vi "SS2 Live_Download Multiple SS2 Images_v3.vi"(4 "# 8-bit Images (1)":i32=1, 5 "Image ROI Information":T2, 6 "Buffer Size (#8-bit Images)":i32, 7 "SS2 Live Gate Data Q Name":string="SS2 Live Gate Data Q", 8 "Error In":errorcluster, 9 "Image Binning Options":T1={"Use Image Binning"=FALSE, "X Bin"=1, "Y Bin"=1} {"Y Bin" min=1; "X Bin" min=1}, 10 "Display Image":T3, 11 "Device Refnum":refnum<k24>) -> (0 "Error Out":errorcluster, 1 "8-bit Image Count":i32, 2 "Display Image":T3)   [LabVIEW 2019]
uses:
  C:/UCLA Thinkpad Google Drive/LabVIEW 2019 SP1/builds/SS2 Live Distribution/Opal Kelly/C# Wrapper/libFrontPanel-csharp.dll
  Opal Kelly/C# Wrapper/libFrontPanel-csharp.dll
  <vilib>/vision/Image Controls.llb/IMAQ Image.ctl
  SS2 Live_Image ROI Information.ctl
  Phasor/Image Binning Options.ctl
  8f499a87-0ce6-40db-98f3-8f764b7e409e.vi
  8d2e2152-5180-46c7-ad9e-0233ef769053.vi
  <vilib>/Utility/High Resolution Relative Seconds.vi
  <vilib>/Utility/error.llb/Error Cluster From Error Code.vi
  <vilib>/ErrorRing/Error Ring.xnode
  Opal Kelly/C# Wrapper/okFrontPanelC#Wrapper.lvlib
  <vilib>/vision/NI_Vision_Development_Module.lvlib
  Notebook/Notebook.lvlib
  Rich Text Box/Rich Text Box.lvlib
panel:
  out "ReadFromBlockPipeout Error":errorcluster
  out "Activate Trigger Error Out":errorcluster
  out "Timeout error":errorcluster
  out "CPU/8-bit Gate":dbl
  in  "Discard First Image":bool
  in  "Block Size":i32=-1
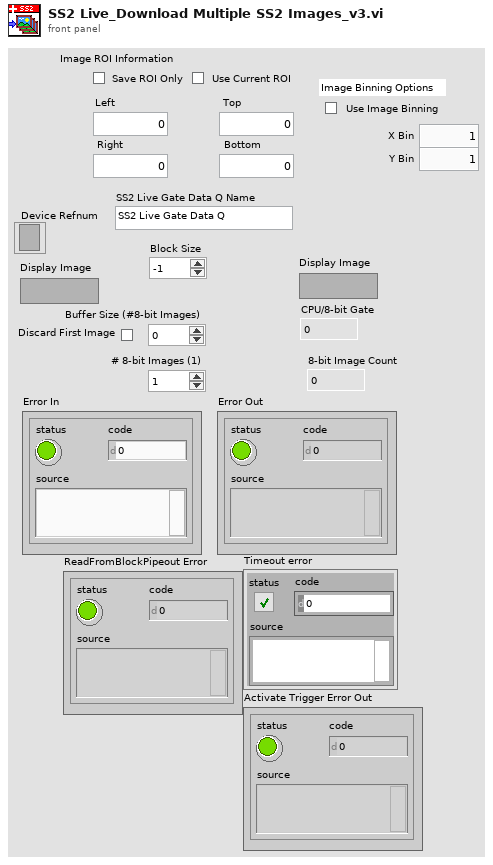
[diagram p1: front panel]
types:
  T1 = typedef "Image Binning Options.ctl" = cluster{"Use Image Binning":bool, "X Bin":i32, "Y Bin":i32}
  T2 = typedef "SS2 Live_Image ROI Information.ctl" = cluster{"Save ROI Only":bool, "Left":u16, "Top":u16, "Right":u16, "Bottom":u16, "Use Current ROI":bool}
  T3 = typedef "IMAQ Image.ctl" = refnum<image>
  T4 = typedef "Image Type" = u32
  T5 = typedef "Rich Text Box.lvlib/Text Formatting.ctl" = cluster{"Font":string, "Text Color":T6, "Text Background Color":T6, "Text Style":enum16{"Regular", "Bold", "Italic", "Underline", "Strikeout"}, "Font Size (Points)":dbl, "Text Alignment":i32}
  T6 = typedef "Rich Text Box.lvlib/Text Colors.ctl" = enum16{"Unchanged", "Black", "Blue", "Gray", "Green", "Red", "White"}
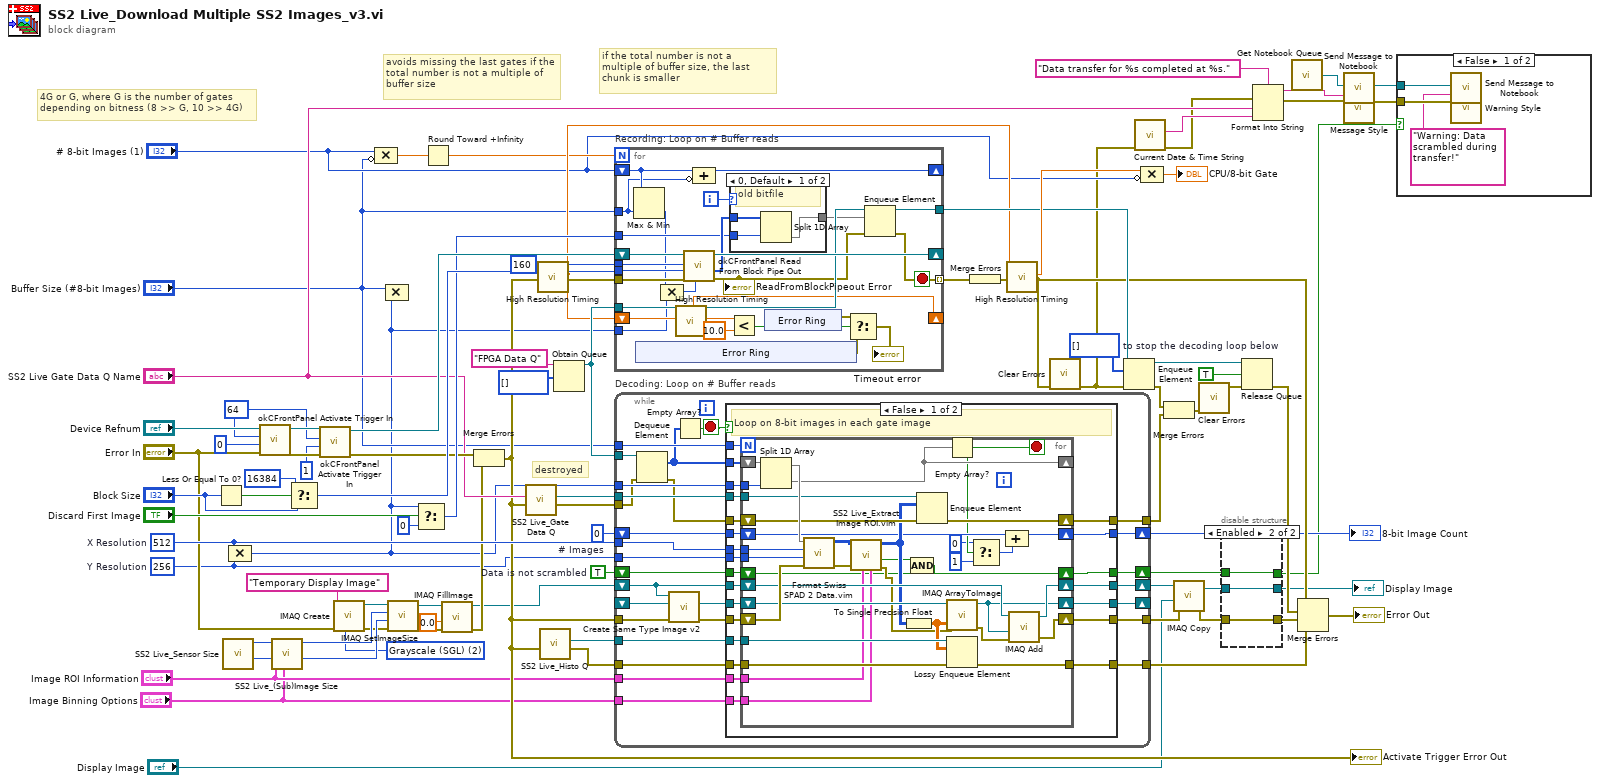
[diagram p0: block diagram]
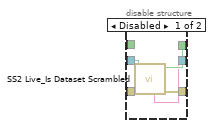
[diagram p2: hidden frame]
diagram:
  w2 = TRUE  # Data is not scrambled
  w21 = T4 2 items=["Grayscale (U8)", "Grayscale (I16)", "Grayscale (SGL)", "Complex (CSG)", "RGB (U32)", "HSL (U32)", "RGB (U64)", "Grayscale (U16)"] ("Image Type")
  w59 = u8[] []  # to stop the decoding loop below
  w61 = 0  # # Images
  w3 = 256  # Y Resolution
  w76 = 512  # X Resolution
  w83 = 64 ("Endpoint Addr")
  # "destroyed"
  # "if the total number is not a multiple of buffer size, the last chunk is smaller"
  # "avoids missing the last gates if the total number is not a multiple of buffer size"
  # "4G or G, where G is the number of gates\ndepending on bitness (8 >> G, 10 >> 4G)"
  n1 = Less Or Equal To 0?(x="Block Size") -> (x <= 0?=w81:bool)
  n2 = call "SS2 Live_Sensor Size.vi"() -> ("Y size"=w22:i32, "X size"=w23:i32)  [unwired: 10 in]
  n3 = Compound Arithmetic op=MULTIPLY(w76, w3) -> (w12:i32)
  n4 = call "okCFrontPanel Activate Trigger In.vi"("Error In"="Error In", "Bit"=0, "Endpoint Addr"=w83, "okCFrontPanel Refnum"="Device Refnum") -> ("Error Out"=w85:errorcluster, "okCFrontPanel Refnum"=w84:refnum<k24>)  [unwired: 6 in]
  n5 = call "SS2 Live_(Sub)Image Size.vi"("Image Binning Options"="Image Binning Options", "Image Information"="Image ROI Information", "# Pixel Y in"=w22, "# Pixel X in"=w23) -> ("# Pixel Y out"=w39:i32, "# Pixel X out"=w40:i32)  [unwired: 6 in]
  n6 = Select(t=16384, s=w81, f="Block Size") -> (s? t:f=w66:i32)
  n7 = call "okCFrontPanel Activate Trigger In.vi"("Error In"=w85, "Bit"=1, "Endpoint Addr"=w83, "okCFrontPanel Refnum"=w84) -> ("Error Out"=w55:errorcluster, "okCFrontPanel Refnum"=w67:refnum<k24>)  [unwired: 6 in]
  n8 = call "IMAQ Create"("Image Name"="Temporary Display Image", "Image Type"=w21, "error in (no error)"="Error In") -> ("New Image"=w34:T3, "error out"=w36:errorcluster)  [unwired: 2 in]
  n9 = Compound Arithmetic op=MULTIPLY("# 8-bit Images (1)", invert "Buffer Size (#8-bit Images)") -> (w19:dbl)
  n10 = Compound Arithmetic op=MULTIPLY("Buffer Size (#8-bit Images)", w12) -> ()  [unwired: 1 out]
  n11 = call "IMAQ SetImageSize"("error in (no error)"=w36, "Y Resolution"=w39, "X Resolution"=w40, "Image"=w34) -> ("error out"=w32:errorcluster, "Image Out"=w33:T3)  [unwired: 1 in]
  n12 = Select(t=w12, s="Discard First Image", f=0) -> (s? t:f=w65:i32)
  n13 = Round Toward +Infinity(x=w19) -> (ceil(x): smallest int >= x=w20:dbl)
  n14 = call "IMAQ FillImage"("error in (no error)"=w32, "Pixel Value (U8, U16, I16, Float)"=sgl 0.0, "Image"=w33) -> ("error out"=w31:errorcluster, "Image Out"=w30:T3)  [unwired: 7 in]
  n15 = Merge Errors(w55, w31) -> (w41:errorcluster)
  "Activate Trigger Error Out" <- w41
  n16 = call "SS2 Live_Gate Data Q.vi"("error in (no error)"=w41, "SS2 Live Gate Data Q Name"="SS2 Live Gate Data Q Name") -> ("error out"=w64:errorcluster, "SS2 Live Gate Data Q"=w77:refnum<queue>)  [unwired: 4 in]
  n17 = call "High Resolution Timing.vi"("Error In"=w41) -> ("elapsed (relative) seconds"=w48:dbl, "Error Out"=w54:errorcluster)  [unwired: 16 in, 1 out]
  n18 = call "SS2 Live_Histo Q.vi"("error in (no error)"=w41) -> ("error out"=w74:errorcluster, "SS2 Live Histo Q"=w75:refnum<queue>)  [unwired: 5 in]
  n19 = Obtain Queue(name (unnamed)="FPGA Data Q", element data type=u8[] [] ("BYTEARRAY")) -> (queue out=w50:refnum<queue>)  [unwired: 3 in, 2 out]
  n20 = for "Recording: Loop on # Buffer reads" {
    N: w20 -> [_]
    tunnel: 160 ("Endpoint Addr") -> [w113]
    shift-right: [w111] -> _
    shift-left: w67 -> [w112]
    tunnel: w66 -> [w108]
    tunnel: w65 -> [w93]
    tunnel: w50 -> [w107]
    tunnel: w54 -> [w94]
    tunnel: [w104] -> w53 mode=indexing
    tunnel: [w103] -> w49
    shift-right: [w99] -> _
    shift-left: w48 -> [w102]
    shift-right: [w92] -> _
    shift-left: "# 8-bit Images (1)" -> [w91]
    tunnel: "Buffer Size (#8-bit Images)" -> [w90]
    tunnel: w12 -> [w88]
    i -> [w109]
    stop <- w104 stop-if-true
    n21 = Max & Min(x=w91, y=w90) -> (min(x,y)=w89:i32)  [unwired: 1 out]
    n22 = xnode "Error Ring"() -> ("error out"=w97:errorcluster)
    n23 = Compound Arithmetic op=MULTIPLY(w89, w88) -> (w87:i32)
    n24 = call "High Resolution Timing.vi"("relative seconds (NaN)"=w102) -> ("relative seconds"=w99:dbl, "elapsed (relative) seconds"=w101:dbl)  [unwired: 16 in, 1 out]
    n25 = call "okCFrontPanel Read From Block Pipe Out.vi"("Length"=w87, "Error In"=w94, "Block Size"=w108, "Endpoint Addr"=w113, "okCFrontPanel Refnum"=w112) -> ("Error Out"=w105:errorcluster, "BYTEARRAY"=w110:u8[], "okCFrontPanel Refnum"=w111:refnum<k24>)  [unwired: 4 in]
    "ReadFromBlockPipeout Error" <- w105
    n26 = Compound Arithmetic op=ADD(w91, invert w90) -> (w92:i32)
    n27 = Less?(x=w101, y=10.0) -> (x < y?=w98:bool)
    n28 = case shown="0, Default" w109 {
      tunnel: w110 -> [w121 w122]
      tunnel: w93 -> [w120 _]
      tunnel: [w119 w122] -> w106
      frame 0, Default {
        # "old bitfile"
        n29 = Split 1D Array(array=w121, index=w120) -> (second subarray=w119:u8[])  [unwired: 1 out]
      }
      frame 1 {
      }
    }
    n30 = xnode "Error Ring"() -> ("error out"=w96:errorcluster)
    n31 = Select(t=w96, s=w98, f=w97) -> (s? t:f=→"Timeout error":errorcluster)
    n32 = Enqueue Element(queue=w107, element=w106, error in (no error)=w105) -> (queue out=w103:refnum<queue>, error out=w104:errorcluster)  [unwired: 1 in, 1 out]
  }
  n33 = while "Decoding: Loop on # Buffer reads" {
    tunnel: w3 -> [w150]
    tunnel: w76 -> [w149]
    tunnel: w41 -> [w142]
    tunnel: "Buffer Size (#8-bit Images)" -> [w148]
    tunnel: w12 -> [w147]
    shift-right: [w133] -> _
    shift-left: _ -> [w145]
    tunnel: [w146] -> w27
    tunnel: w77 -> [w140]
    tunnel: w64 -> [w131]
    tunnel: [w139] -> w60
    tunnel: w75 -> [w138]
    tunnel: w74 -> [w137]
    tunnel: [w136] -> w73
    shift-right: [w135] -> w28
    shift-left: w30 -> [w144]
    tunnel: w50 -> [w132]
    shift-right: [w141] -> w38
    shift-left: w61 -> [w127]
    tunnel: "Image ROI Information" -> [w126]
    tunnel: "Image Binning Options" -> [w125]
    shift-right: [w124] -> w5
    shift-left: w2 -> [w123]
    stop <- w128 stop-if-true
    n34 = Dequeue Element(queue=w132, error in (no error)=w131) -> (element=w129:u8[], error out=w130:errorcluster)  [unwired: 1 in, 2 out]
    n35 = call "Create Same Type Image v2.vi"("error in (no error)"=w142, "Image Dst"=w145, "Image Src"=w144) -> ("error out"=w143:errorcluster, "Image Dst"=w134:T3)  [unwired: 6 in, 1 out]
    n36 = Empty Array?(array=w129) -> (empty?=w128:bool)
    n37 = case shown="False" w128 {
      tunnel: w150 -> [w173 _]
      tunnel: w149 -> [w172 _]
      tunnel: w148 -> [w171 _]
      tunnel: w147 -> [w170 _]
      tunnel: [w169 w211] -> w146
      tunnel: w144 -> [w168 w213]
      tunnel: w143 -> [w167 w211]
      tunnel: [w154 w214] -> w141
      tunnel: w140 -> [w166 _]
      tunnel: [w165 w215] -> w139
      tunnel: w138 -> [w164 _]
      tunnel: w137 -> [w163 w210]
      tunnel: [w162 w210] -> w136
      tunnel: [w161 w213] -> w135
      tunnel: w134 -> [w160 w212]
      tunnel: [w159 w212] -> w133
      tunnel: w130 -> [w158 w215]
      tunnel: w129 -> [w157 _]
      tunnel: w127 -> [w155 w214]
      tunnel: w126 -> [w156 _]
      tunnel: w125 -> [w153 _]
      tunnel: [w151 w209] -> w124
      tunnel: w123 -> [w152 w209]
      frame False {
        # "Loop on 8-bit images in each gate image"
        n38 = for {
          N: w171 -> [_]
          tunnel: w173 -> [w208]
          tunnel: w172 -> [w207]
          shift-right: [w199] -> w169
          shift-left: w167 -> [w206]
          shift-right: [w198] -> _
          shift-left: w157 -> [w205]
          tunnel: w170 -> [w203]
          tunnel: w166 -> [w197]
          shift-right: [w195] -> w165
          shift-left: w158 -> [w196]
          tunnel: w164 -> [w194]
          tunnel: w163 -> [w193]
          tunnel: [w192] -> w162
          shift-right: [w190] -> w161
          shift-left: w168 -> [w201]
          shift-right: [w189] -> w159
          shift-left: w160 -> [w202]
          tunnel: w156 -> [w178]
          shift-right: [w183] -> w154
          shift-left: w155 -> [w184]
          tunnel: w153 -> [w177]
          shift-right: [w174] -> w151
          shift-left: w152 -> [w175]
          stop <- w182 stop-if-true
          n39 = Split 1D Array(array=w205, index=w203) -> (first subarray=w204:u8[], second subarray=w198:u8[])
          n40 = call "Format Swiss SPAD 2 Data.vim"("Error In"=w206, "Y Resolution"=w208, "X Resolution"=w207, "Flattened Image"=w204) -> ("Error Out"=w187:errorcluster, "Image out"=w188:u8[][])  [unwired: 6 in]
          n41 = call "SS2 Live_Extract Image ROI.vim"("Image Binning Options"=w177, "Image Information"=w178, "Error In"=w187, "Image in"=w188) -> ("Error Out"=w186:errorcluster, "Data is not scrambled"=w176:bool, "Image out"=w185:u8[][])  [unwired: 5 in]
          n42 = To Single Precision Float(number=w185) -> (single precision float=w191:sgl[][])
          n43 = Compound Arithmetic op=AND(w176, w175) -> (w174:bool)
          n44 = Enqueue Element(queue=w197, element=w185, error in (no error)=w196) -> (error out=w195:errorcluster)  [unwired: 1 in, 2 out]
          n45 = Empty Array?(array=w198) -> (empty?=w182:bool)
          n46 = call "IMAQ ArrayToImage"("Image Pixels (Float)"=w191, "error in (no error)"=w186, "Image"=w202) -> ("error out"=w200:errorcluster, "Image Out"=w189:T3)  [unwired: 7 in]
          n47 = Lossy Enqueue Element(queue=w194, element=w191, error in (no error)=w193) -> (error out=w192:errorcluster)  [unwired: 3 out]
          n48 = Select(t=0 ("value"), s=w182, f=1) -> (s? t:f=w181:i32)
          n49 = Compound Arithmetic op=ADD(w184, w181) -> (w183:i32)
          n50 = call "IMAQ Add"("Image Src A"=w201, "Image Src B"=w189, "error in (no error)"=w200) -> ("Image Dst Out"=w190:T3, "error out"=w199:errorcluster)  [unwired: 4 in]
        }
      }
      frame True {
        # "No data: end"
      }
    }
  }
  "8-bit Image Count" <- w38
  n51 = Merge Errors(w53) -> (w51:errorcluster)
  n52 = call "High Resolution Timing.vi"("relative seconds (NaN)"=w48, "Error In"=w51) -> ("elapsed (relative) seconds"=w52:dbl, "Error Out"=w42:errorcluster)  [unwired: 15 in, 1 out]
  n53 = call <vilib>:"Clear Errors.vi"("error in (no error)"=w42) -> ("error out"=w15:errorcluster)  [unwired: 5 in, 1 out]
  n54 = Enqueue Element(queue=w49, element=w59, error in (no error)=w15) -> (queue out=w56:refnum<queue>, error out=w57:errorcluster)  [unwired: 1 in, 1 out]
  n55 = call "Current Date & Time String.vi"("Error In"=w15) -> ("Error Out"=w14:errorcluster, "time string"=w16:string)  [unwired: 8 in, 1 out]
  n56 = Compound Arithmetic op=MULTIPLY(w52, invert "# 8-bit Images (1)") -> (→"CPU/8-bit Gate":dbl)
  n57 = Merge Errors(w57, w60) -> (w58:errorcluster)
  n58 = call "IMAQ Copy"("error in (no error)"=w27, "Image Dst"="Display Image", "Image Src"=w28) -> ("error out"=w11:errorcluster, "Image Dst Out"=w9:T3)  [unwired: 3 in]
  "Display Image" <- w9
  n59 = call <vilib>:"Clear Errors.vi"("error in (no error)"=w58) -> ("error out"=w1:errorcluster)  [unwired: 5 in, 1 out]
  n60 = disable-structure shown="Enabled" {
    disable-tunnel: w11 -> [w220 w222]
    disable-tunnel: [w219 w222] -> w10
    disable-tunnel: w9 -> [w218 w223]
    disable-tunnel: [w217 w221] -> w6
    disable-tunnel: [w216 w223] -> _
    disable-tunnel: w5 -> [_ w221]
    frame Disabled {
      n61 = call "SS2 Live_Is Dataset Scrambled.vi"("Error In"=w220, "Refnum in"=w218) -> ("Error Out"=w219:errorcluster, "SS2 image is scrambled"=w217:bool, "Warning"=w216:string)  [unwired: 4 in, 3 out]
    }
    frame Enabled {
    }
  }
  n62 = Release Queue(queue=w56, force destroy? (F)=TRUE, error in (no error)=w1) -> (error out=w43:errorcluster)  [unwired: 2 out]
  n63 = Format Into String(format string="Data transfer for %s completed at %s.", error in=w14, "SS2 Live Gate Data Q Name", w16) -> (resulting string=w44:string, error out=w17:errorcluster)  [unwired: 1 in]
  n64 = call "Get Notebook Queue.vi"() -> ("Notebook Queue"=w8:refnum<queue>)  [unwired: 9 in]
  n65 = Merge Errors(w42, w43, w10, w73) -> (→"Error Out":errorcluster)
  n66 = call "Message Style.vi"() -> ("Message Formatting"=w47:T5)
  n67 = call "Send Message to Notebook.vi"("Notebook Queue"=w8, "Message"=w44, "Error In"=w17, "Text Formatting"=w47) -> ("Error Out"=w7:errorcluster)  [unwired: 15 in]
  n68 = case shown="False" w6 {
    tunnel: w8 -> [w227 _]
    tunnel: w7 -> [w226 _]
    frame False {
      n69 = call "Warning Style.vi"() -> ("Error Formatting"=w225:T5)
      n70 = call "Send Message to Notebook.vi"("Notebook Queue"=w227, "Message"="Warning: Data scrambled during transfer!" ("format string"), "Error In"=w226, "Text Formatting"=w225) -> ()  [unwired: 15 in, 1 out]
    }
    frame True {
    }
  }
